vi "close.vi"(8 "error in (no error)":errorcluster, 11 "HamegHMPSupply in":refnum<class "HamegHMPSupply.lvclass">) -> (0 "error out":errorcluster)   [LabVIEW 2011, in "Hardware.lvlib" / "Channels.lvlib" / "HamegHMPSupply.lvclass"]
doc: "Closes the analog output device."
uses:
  HamegHMPSupply.lvclass
  HamegHMPSupply.lvclass/HamegHMPSupply.ctl
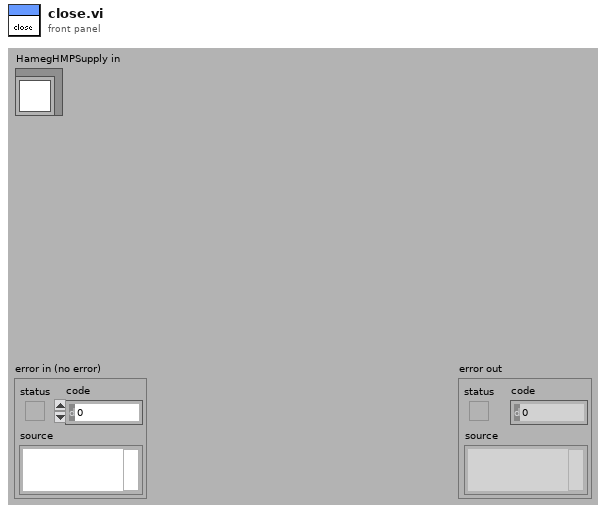
[diagram p1: front panel]
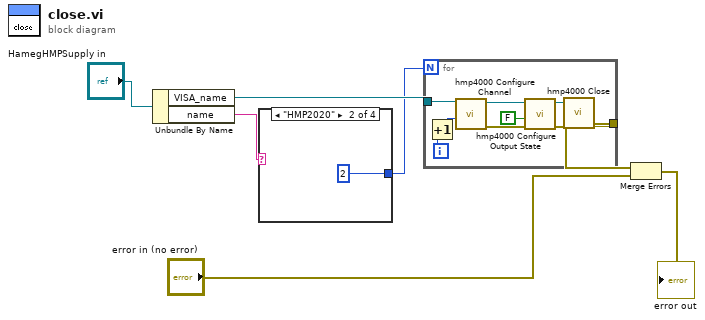
[diagram p0: block diagram]
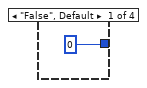
[diagram p2: hidden frame]
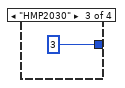
[diagram p3: hidden frame]
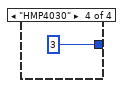
[diagram p4: hidden frame]
diagram:
  n1 = Unbundle By Name("HamegHMPSupply in") -> ("VISA_name"=w3:refnum<visa-resource-name>, "name"=w2:string)
  n2 = case shown="\"HMP2020\"" w2 {
    tunnel: [0 2 3 3] -> w1
    frame "False", Default {
    }
    frame "HMP2020" {
    }
    frame "HMP2030" {
    }
    frame "HMP4030" {
    }
  }
  n3 = for {
    N: w1 -> [_]
    tunnel: [w20] -> w6
    tunnel: w3 -> [w16]
    i -> [w13]
    n4 = Increment(x=w13) -> (x+1=w12:i32)
    n5 = call <instrlib>:"hmp4000 Configure Channel.vi"("Channel (Channel 1)"=w12, "VISA resource name"=w16) -> ("error out"=w14:errorcluster, "VISA resource name out"=w15:refnum<visa-resource-name>)  [unwired: 8 in]
    n6 = call <instrlib>:"hmp4000 Configure Output State.vi"("error in (no error)"=w14, "Output State (Off)"=FALSE, "VISA resource name"=w15) -> ("error out"=w18:errorcluster, "VISA resource name out"=w19:refnum<visa-resource-name>)  [unwired: 7 in]
    n7 = call <instrlib>:"hmp4000 Close.vi"("error in (no error)"=w18, "VISA resource name"=w19) -> ("error out"=w20:errorcluster)  [unwired: 9 in]
  }
  n8 = Merge Errors(w6, "error in (no error)") -> (→"error out":errorcluster)
